vi "Signal.StartBit.Calculate.vi"(10 "Length":u32=22, 11 "Byte Order":u32(ring) items=["Little Endian", "Big Endian"]) -> (3 "Start Bit":u32)   [LabVIEW 2019, in "Diagnostics Addon System Explorer.lvlib"]
uses:
  Diagnostics Addon System Explorer.lvlib
  Shared/Types/Signal.ctl
  Shared/Diagnostics Addon Shared.lvlib
panel:
  in  "Signal2":T1 {"Byte Order" items=["Little Endian", "Big Endian"]; "Data Type" items=["Signed", "Unsigned", "IEEE Float"]}
  in  "Signal1":T1 {"Byte Order" items=["Little Endian", "Big Endian"]; "Data Type" items=["Signed", "Unsigned", "IEEE Float"]}
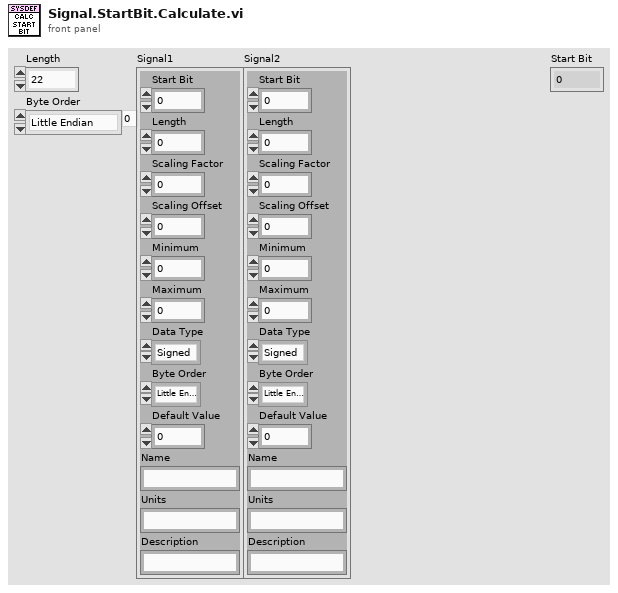
[diagram p1: front panel]
types:
  T1 = typedef "Diagnostics Addon Shared.lvlib/Signal.ctl" = cluster{"Start Bit":u32, "Length":u32, "Scaling Factor":dbl, "Scaling Offset":dbl, "Minimum":dbl, "Maximum":dbl, "Data Type":u32, "Byte Order":u32, "Default Value":dbl, "Name":string, "Units":string, "Description":string}
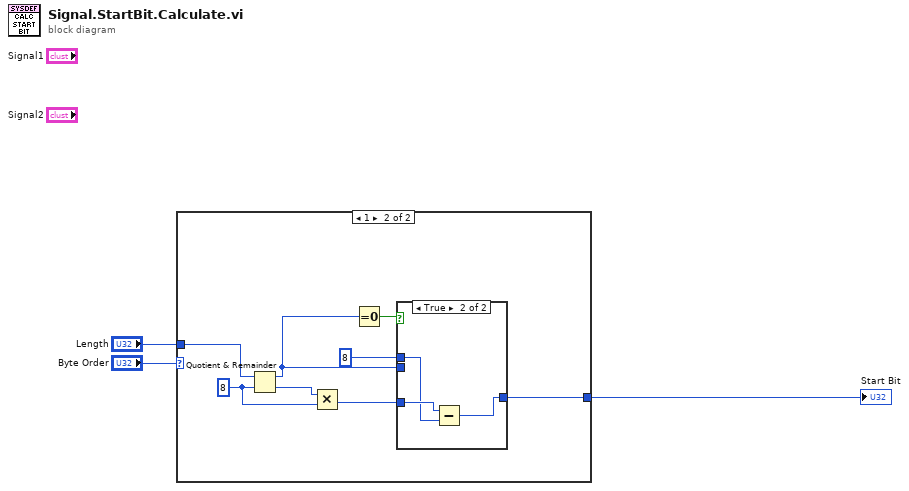
[diagram p0: block diagram]
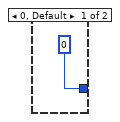
[diagram p2: hidden frame]
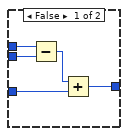
[diagram p3: hidden frame]
diagram:
  n1 = case shown="1" "Byte Order" {
    tunnel: "Length" -> [_ w5]
    tunnel: [0 w8] -> w3
    frame 0, Default {
    }
    frame 1 {
      w11 = u32 8 ("y")
      n2 = Quotient & Remainder(x=w5, y=w11) -> (x-y*floor(x/y)=w7:u32, floor(x/y)=w12:u32)
      n3 = Multiply(x=w12, y=w11) -> (x*y=w9:u32)
      n4 = Equal To 0?(x=w7) -> (x = 0?=w6:bool)
      n5 = case shown="True" w6 {
        tunnel: 8 ("x") -> [w17 w19]
        tunnel: w9 -> [w15 w20]
        tunnel: [w14 w18] -> w8
        tunnel: w7 -> [w13 _]
        frame False {
          n6 = Subtract(x=w17, y=w13) -> (x-y=w16:u32)
          n7 = Add(x=w16, y=w15) -> (x+y=w14:u32)
        }
        frame True {
          n8 = Subtract(x=w20, y=w19) -> (x-y=w18:u32)
        }
      }
    }
  }
  "Start Bit" <- w3
